vi "PXIe_2584.vi"   [LabVIEW 2021]
uses:
  <instrlib>/niSwitch/niSwitch.llb/niSwitch Topologies.ctl
  <instrlib>/niSwitch/niSwitch.llb/niSwitch Connect Channels (Single).vi
types:
  T1 = typedef "niSwitch Topologies.ctl" = string
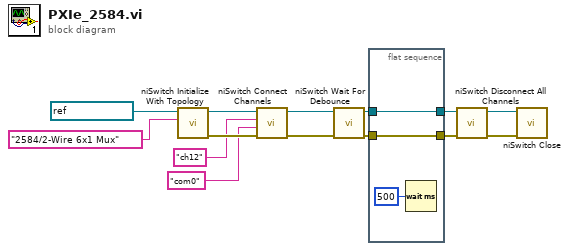
[diagram p0: block diagram]
diagram:
  n1 = call <instrlib>:"niSwitch Initialize With Topology.vi"("topology name"=T1 "2584/2-Wire 6x1 Mux", "resource name"=refnum<k15> "PXI1Slot10") -> ("error out"=w11:errorcluster, "instrument handle out"=w12:refnum<k15>)  [unwired: 8 in]
  n2 = call-poly <instrlib>:"niSwitch Connect Channels.vi"("error in (no error)"=w11, "channel 2"="com0", "channel 1"="ch12", "instrument handle"=w12) -> ("error out"=w10:errorcluster, "instrument handle out"=w9:refnum<k15>)  [unwired: 6 in]
  n3 = call <instrlib>:"niSwitch Wait For Debounce.vi"("error in (no error)"=w10, "instrument handle"=w9) -> ("error out"=w6:errorcluster, "instrument handle out"=w8:refnum<k15>)  [unwired: 8 in]
  n4 = flat-sequence {
    tunnel: w8 -> [w17]
    tunnel: [w17] -> w7
    tunnel: w6 -> [w16]
    tunnel: [w16] -> w5
    frame #0 {
      n5 = Wait (ms)(milliseconds to wait=u32 500) -> ()  [unwired: 1 out]
    }
  }
  n6 = call <instrlib>:"niSwitch Disconnect All Channels.vi"("error in (no error)"=w5, "instrument handle"=w7) -> ("error out"=w4:errorcluster, "instrument handle out"=w3:refnum<k15>)  [unwired: 8 in]
  n7 = call <instrlib>:"niSwitch Close.vi"("error in (no error)"=w4, "instrument handle"=w3) -> ()  [unwired: 9 in, 1 out]
